vi "SimpleFreerun.vi"() -> ()   [LabVIEW 2010]
uses:
  Motion/EnableSingle.vi
  Motion/FreerunSingle.vi
  Motion/AbortSingle.vi
  Motion/DisableSingle.vi
panel:
  in  "milliseconds to run":u32=1000
  in  "return immediately":bool
  out "Position":string
  in  "Speed":dbl=5000.0
  in  "Axis Name":string="X"
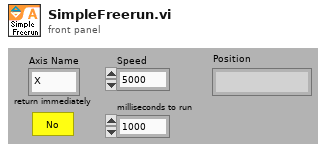
[diagram p1: front panel]
types:
  T1 = typedef "ControllerDiagPacket.ctl" = cluster{"Number of Diag Packets":i32, "Axes":T2[], "error":errorcluster}
  T2 = typedef "AxisDiagPacket.ctl" = cluster{"Axis Name":string, "Analog Input 0":dbl, "Analog Input 1":dbl, "Axis Fault (num)":i32, "Axis Fault (str)":string, "Axis Fault (bits)":cluster{"AmplifierFault":bool, "AmplifierTemperatureFault":bool, "CcwEndOfTravelLimitFault":bool, "CcwSoftwareLimitFault":bool, "CommunicationLostFault":bool, "CwEndOfTravelLimitFault":bool, "CwSoftwareLimitFault":bool, "EmergencyStopFault":bool, "EncoderFault":bool, "ExternalFault":bool, "FeedbackScalingFault":bool, "GantryMisalignFault ":bool, "HallSensorFault":bool, "InPositionTimeoutFault":bool, "MarkerSearchFault":bool, "MaxVelocityCommandFault":bool, "MissedInterruptFault":bool, "MotorTemperatureFault":bool, "None":bool, "OverCurrentFault":bool, "PositionErrorFault":bool, "PositionFeedbackFault":bool, "PowerSupplyFault":bool, "ProbeInputFault":bool, "SafeZoneFault":bool, "VelocityErrorFault":bool, "VelocityFeedbackFault":bool, "VoltageClampFault":bool}, "Axis Status (num)":i32, "Axis Status (str)":string, "Axis Status (bits)":cluster{"BacklashActive":bool, "CalibrationEnabled1D":bool, "CalibrationEnabled2D":bool, "CommandValid":bool, "DriveAbortPending":bool, "DrivePending":bool, "Enabling":bool, "GainMappingEnabled":bool, "GantryAligned":bool, "GantryRealigning":bool, "Homed":bool, "Homing":bool, "IFOVEnabled":bool, "JogGenerating":bool, "Jogging":bool, "JoystickControl":bool, "MasterSlaveControl":bool, "MotionBlocked":bool, "MotionClamped":bool, "MoveDone":bool, "None":bool, "NotVirtual":bool, "Profiling":bool, "Stability0":bool, "Stability1":bool, "TrajectoryFiltering":bool, "WaitDone":bool}, "Current Command":sgl, "Current Error":sgl, "Current Feedback":sgl, "Digital Inputs":i32, "Digital Outputs":i32, "Drive Status":i32, "Drive Status (str)":string, "Drive Status (bits)":cluster{"AccelerationPhase":bool, "AutofocusActive":bool, "BrakeOutput":bool, "CcwEndOfTravelLimitInput":bool, "CosineEncoderError":bool, "CurrentClamp":bool, "CwEndOfTravelLimitInput":bool, "DecelerationPhase":bool, "DualLoopActive":bool, "EmergencyStopInput":bool, "Enabled":bool, "EncoderClipping":bool, "GalvoCalibrationEnabled":bool, "GalvoPowerCorrection":bool, "HallAInput":bool, "HallBInput":bool, "HallCInput":bool, "HighResolutionMode":bool, "HomeLimitInput":bool, "InPosition":bool, "InPosition2":bool, "MarkerInput":bool, "MarkerLatch":bool, "MoveActive":bool, "NoMotorSupply":bool, "None":bool, "PowerLimiting":bool, "ProgrammingFlash":bool, "ProgrammingMXH":bool, "PSOHaltLatch":bool, "ServoControl":bool, "SineEncoderError":bool}, "Position Feedback Auxiliary":dbl, "Position Command":dbl, "Position Error":dbl, "Position Feedback":dbl, "Program Position Command":dbl, "Program Position Error":dbl, "Program Position Feedback":dbl, "Velocity Command":dbl, "Velocity Error":dbl, "Velocity Feedback":dbl}
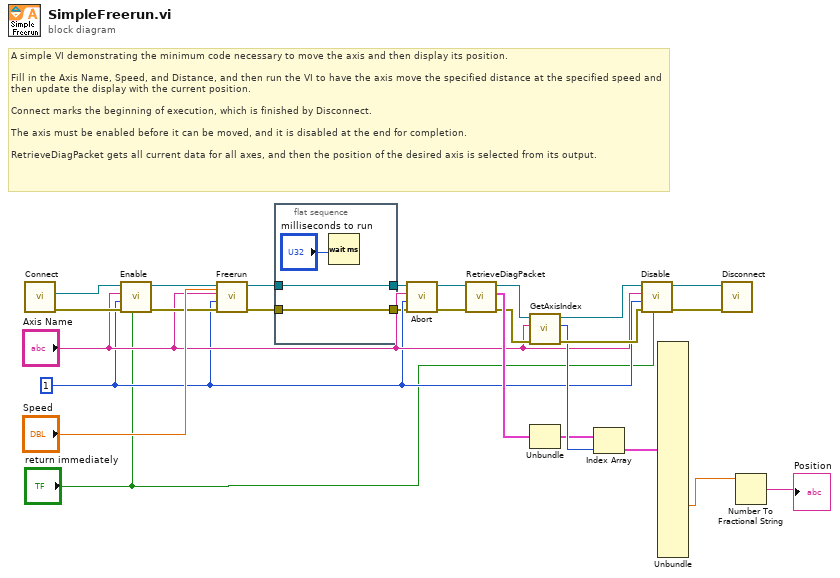
[diagram p0: block diagram]
diagram:
  w6 = 1 ("taskNumber")
  # "A simple VI demonstrating the minimum code necessary to move the axis and then display its position.\n\nFill in the Axis Name, Speed, and Distance, and then run the VI to have the axis move the specified distance at the specified speed and then update the display with the current position.\n\nConnect marks the beginning of execution, which is finished by Disconnect.\n\nThe axis must be enabled before it can be moved, and it is disabled at the end for completion.\n\nRetrieveDiagPacket gets all current data for all axes, and then the position of the desired axis is selected from its output."
  n1 = call "Connect.vi"() -> ("error out"=w15:errorcluster, "controller"=w16:refnum<k24>)  [unwired: 10 in]
  n2 = call-poly "Enable.vi"("return immediately"="return immediately", "error in (no error)"=w15, "taskId"=w6, "axis name"="Axis Name", "controller in"=w16) -> ("error out"=w14:errorcluster, "controller out"=w13:refnum<k24>)  [unwired: 5 in]
  n3 = call-poly "Freerun.vi"("speed"="Speed", "error in (no error)"=w14, "taskId"=w6, "axis name"="Axis Name", "controller in"=w13) -> ("error out"=w3:errorcluster, "controller out"=w5:refnum<k24>)  [unwired: 5 in]
  n4 = flat-sequence {
    tunnel: w5 -> [w29]
    tunnel: [w29] -> w4
    tunnel: [w28] -> w2
    tunnel: w3 -> [w28]
    frame #0 {
      n5 = Wait (ms)(milliseconds to wait="milliseconds to run") -> ()  [unwired: 1 out]
    }
  }
  n6 = call-poly "Abort.vi"("error in (no error)"=w2, "taskId"=w6, "axis name? (all)"="Axis Name", "controller in"=w4) -> ("error out"=w7:errorcluster, "controller out"=w9:refnum<k24>)  [unwired: 6 in]
  n7 = call "RetrieveDiagPacket.vi"("error in (no error)"=w7, "Controller In"=w9) -> ("error out"=w22:errorcluster, "ControllerDiagPacket"=w24:T1, "Controller Out"=w21:refnum<k24>)  [unwired: 7 in]
  n8 = call "GetAxisIndex.vi"("error in (no error)"=w22, "axis name"="Axis Name", "controller in"=w21) -> ("error out"=w19:errorcluster, "axis index"=w18:i32, "controller out"=w20:refnum<k24>)  [unwired: 6 in]
  n9 = Unbundle(w24) -> ("Axes"=w11:T2[])  [unwired: 2 out]
  n10 = Index Array(array=w11, index=w18) -> (element=w17:T2)
  n11 = call-poly "Disable.vi"("return immediately"="return immediately", "error in (no error)"=w19, "taskId"=w6, "axis name"="Axis Name", "controller in"=w20) -> ("error out"=w26:errorcluster, "controller out"=w12:refnum<k24>)  [unwired: 5 in]
  n12 = Unbundle(w17) -> ("Position Feedback"=w10:dbl)  [unwired: 26 out]
  n13 = call "Disconnect.vi"("error in (no error)"=w26, "controller"=w12) -> ()  [unwired: 9 in, 1 out]
  n14 = Number To Fractional String(number=w10) -> (F-format string=→"Position":string)  [unwired: 3 in]
